vi "Speed graph window.vi"() -> ()   [LabVIEW 2020]
uses:
  Typedefs/Notifier Function.ctl
  Global Variables/General Globals.vi
  Globals/Encoder globals.vi
panel:
  out "Logging":bool
  out "Encoder disconnected":bool=TRUE
  out "Folder path":path
  out "Update interval":u32 format="Speed update interval: %.0f ms"
  out "Stop":bool
  out "Chart":dbl(graph)
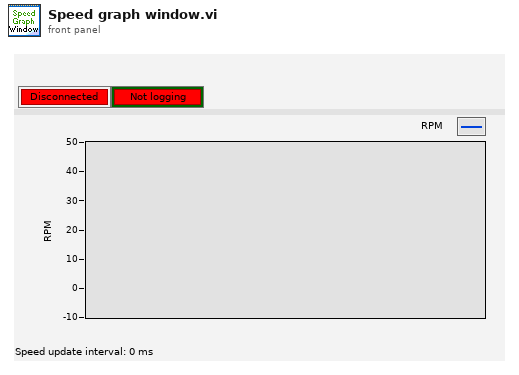
[diagram p1: front panel]
types:
  T1 = typedef "Notifier Function.ctl" = enum16{"Send notifier", "Wait on notification", "Release notifier"}
  T2 = typedef "Speed window notifier data.ctl" = cluster{"Angle (Deg)":dbl, "Data value (rpm)":dbl, "Relative time (uS)":i32, "File path":path, "Logging state":T3}
  T3 = typedef "Speed logging states enum.ctl" = enum16{"Idle", "Open file", "Log", "Close file"}
  T4 = enum32{"Invalid", "Standard", "Closed", "Hidden", "Minimized", "Maximized"}
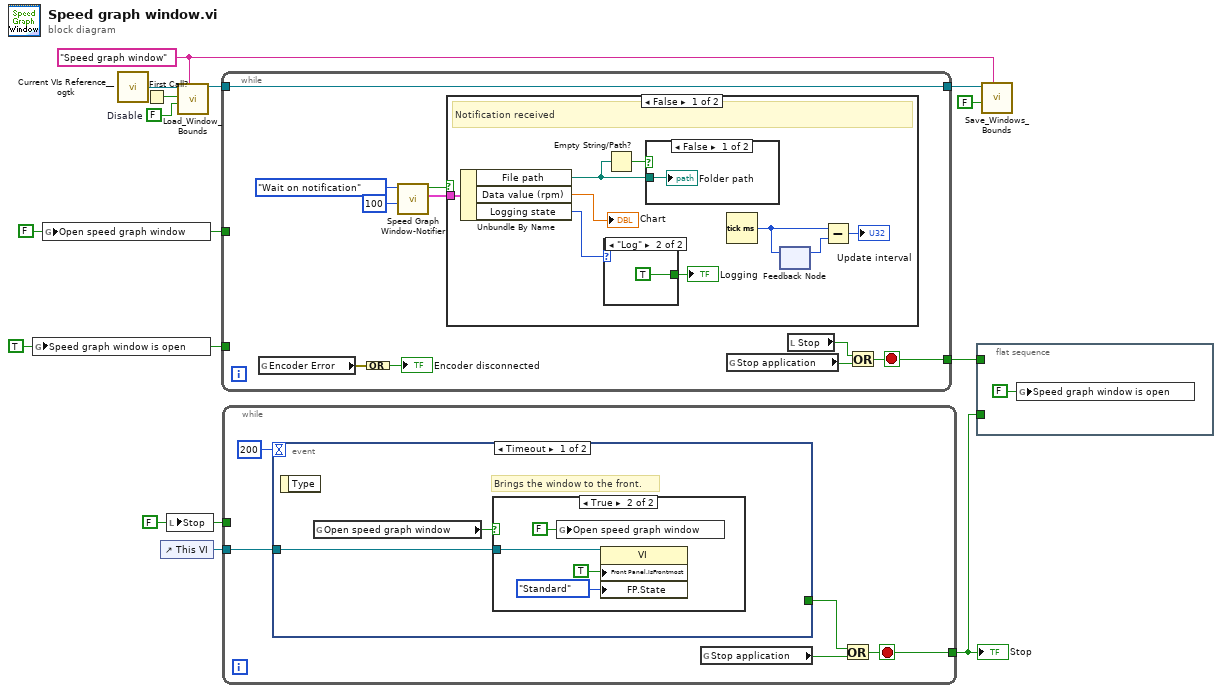
[diagram p0: block diagram]
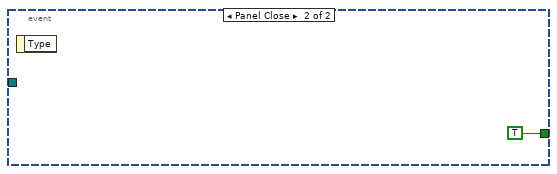
[diagram p3: hidden frame]
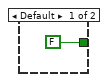
[diagram p4: hidden frame]
diagram:
  w6 = FALSE  # Disable
  w5 = "Speed graph window" ("Window Name (i.e. Key)")
  w11 = TRUE ("Speed graph window is open")
  w12 = FALSE ("Stop")
  w13 = FALSE ("Open speed graph window")
  n1 = global write "General Globals.vi" "Speed graph window is open"(w11) -> ()
  n2 = global write "General Globals.vi" "Open speed graph window"(w13) -> ()
  n3 = call <userlib>:"Current VIs Reference__ogtk.vi"() -> ("Current VI's reference"=w8:refnum<vi>)  [unwired: 5 in]
  n4 = First Call?() -> (First Call?: T/F=w7:bool)
  n5 = control-ref of="This VI"() -> (w1:refnum<vi>)
  n6 = local write "Stop"(w12) -> ()
  n7 = call "Load_Window_Bounds.vi"("Window Name (i.e. Key)"=w5, "Disable"=w6, "First Call"=w7, "Window VI's Ref"=w8) -> ("reference out"=w2:refnum<vi>)  [unwired: 4 in, 3 out]
  n8 = while {
    tunnel: w13 -> [_]
    tunnel: w11 -> [_]
    tunnel: [w17] -> w10
    tunnel: w2 -> [w14]
    tunnel: [w14] -> w3
    stop <- w17 stop-if-true
    n9 = global read "Encoder globals.vi" "Encoder Error"() -> (w16:errorcluster)
    n10 = Compound Arithmetic op=OR(w16) -> (→"Encoder disconnected":bool)
    n11 = call "Speed Graph Window-Notifier.vi"("Timeout waiting in ms (-1)"=100, "Notifier Function"=Notifier_Function."Wait on notification") -> ("Notification data received"=w19:T2, "Timed out waiting"=w22:bool)  [unwired: 7 in, 1 out]
    n12 = case shown="False" w22 {
      tunnel: w19 -> [w29 _]
      frame False {
        # "Notification received"
        n13 = Unbundle By Name(w29) -> ("File path"=w30:path, "Data value (rpm)"=→"Chart":dbl, "Logging state"=w28:T3)
        n14 = case shown="\"Log\"" w28 {
          tunnel: [FALSE TRUE] -> w27
          frame Default {
          }
          frame "Log" {
          }
        }
        "Logging" <- w27
        n15 = Empty String/Path?(string/path=w30) -> (empty?=w31:bool)
        n16 = case shown="False" w31 {
          tunnel: w30 -> [w35 _]
          frame False {
            "Folder path" <- w35
          }
          frame True {
          }
        }
        n17 = Tick Count (ms)() -> (millisecond timer value=w26:u32)
        n18 = feedback #1() -> (w25:u32)  [unwired: 1 in]
        n19 = feedback-in #1(w26) -> ()
        n20 = Subtract(x=w26, y=w25) -> (x-y=→"Update interval":u32)
      }
      frame True {
        # "Timed out waiting"
      }
    }
    n21 = global read "General Globals.vi" "Stop application"() -> (w23:bool)
    n22 = local read "Stop"() -> (w18:bool)
    n23 = Or(x=w18, y=w23) -> (x .or. y?=w17:bool)
  }
  n24 = while {
    tunnel: [w37] -> w9
    tunnel: w12 -> [_]
    tunnel: w1 -> [w36]
    stop <- w37 stop-if-true
    n25 = event shown="[0] Timeout" {
      selector: _ -> [_ _]
      dyn-events: _ -> [_ _]
      timeout: 200 -> [_ _]
      tunnel: [_ TRUE] -> w38
      tunnel: w36 -> [w41 _]
      event Timeout {
        # "Brings the window to the front."
        n26 = event-data() -> ()  [unwired: 1 in, 1 out]
        n27 = global read "General Globals.vi" "Open speed graph window"() -> (w42:bool)
        n28 = case shown="True" w42 {
          tunnel: w41 -> [_ w43]
          frame False {
          }
          frame True {
            n29 = global write "General Globals.vi" "Open speed graph window"(FALSE ("Open speed graph window")) -> ()
            n30 = property class="VI"(reference=w43, "Front Panel.IsFrontmost"=TRUE ("Front Panel Window:Is Frontmost"), "FP.State"=T4."Standard" ("Front Panel Window:State")) -> ()  [unwired: 1 in, 2 out]
          }
        }
      }
      event Panel Close {
        n31 = event-data() -> ()  [unwired: 1 in, 1 out]
      }
    }
    n32 = global read "General Globals.vi" "Stop application"() -> (w40:bool)
    n33 = Or(x=w38, y=w40) -> (x .or. y?=w37:bool)
  }
  "Stop" <- w9
  n34 = flat-sequence {
    tunnel: w10 -> [_]
    tunnel: w9 -> [_]
    frame #0 {
      n35 = global write "General Globals.vi" "Speed graph window is open"(FALSE ("Speed graph window is open")) -> ()
    }
  }
  n36 = call "Save_Windows_Bounds.vi"("Window Name (i.e. Key)"=w5, "Front Panel Window:Open"=FALSE, "Window VI's Ref"=w3) -> ()  [unwired: 8 in, 1 out]
